vi "protocol_combined.vi"() -> ()   [LabVIEW 2015]
uses:
  dxl_x86_c.lvlib/dxl_x86_c.lvlib
panel:
  out "protocol_version2":dbl=2.0
  in  "value : MX (dial)\ngoal position 1":u16(knob)
  in  "ADDR_MX_\nPRESENT_POSITION":u16=36
  in  "ADDR_MX_\nGOAL_POSITION":u16=30
  in  "ADDR_MX_\nTORQUE_ENABLE":u16=24
  out "value : PRO (knob)\npresent position 2":i32(knob) scale=150000.0..-150000.0
  in  "dynamixe2_id":u8=2
  in  "device_name1":string="COM1"
  in  "ADDR_PRO_\nPRESENT_POSITION":u16=611
  in  "ADDR_PRO_\nGOAL_POSITION":u16=596
  in  "ADDR_PRO_\nTORQUE_ENABLE":u16=562
  out "protocol_version1":dbl=1.0
  out "value : MX (knob)\npresent position 1":u16(knob)
  in  "terminate":bool
  out "port_num":i32
  in  "value : PRO (dial)\ngoal position 2":i32(knob) scale=150000.0..-150000.0
  in  "dynamixel1_id":u8=1
  in  "baud_rate":i32=1000000
  # "protocol_combined.vi\n\nCreated on: 2016. 6. 13\nAuthor: Ryu Woon Jung (Leon)\n\n*********     Protocol Combined Example      *********\n\n\nAvailable Dynamixel model on this example : All models using Protocol 1.0 and 2.0\nThis example is designed for using a Dynamixel MX-28, a Dynamixel PRO 54-200 and an USB2DYNAMIXEL\nTo use another Dynamixel model, such as X series, see their details in E-Manual(support.robotis.com) \n   and edit \"numeric control\"s seen left with \"Edit Text\" tool.\nBe sure that properties of Dynamixel MX and PRO are already set as %% MX - ID : 1 / Baudnum : 1 (Baudrate : 1000000) , PRO - ID : 1 / Baudnum : 3 (Baudrate : 1000000)\n\nBe aware that:\nThis example configures two different control tables (especially, if it uses Dynamixel and Dynamixel PRO). It may modify critical Dynamixel parameter on the control table, if Dynamixels have wrong ID.\n\n\n1. Run example by click above \"Run\" button (below \"Edit\" menu).\n2. Drag \"dial\" then you may see the Dynamixel and \"knob\"s rotating\n3. To finish the example, press \"terminate\" button."
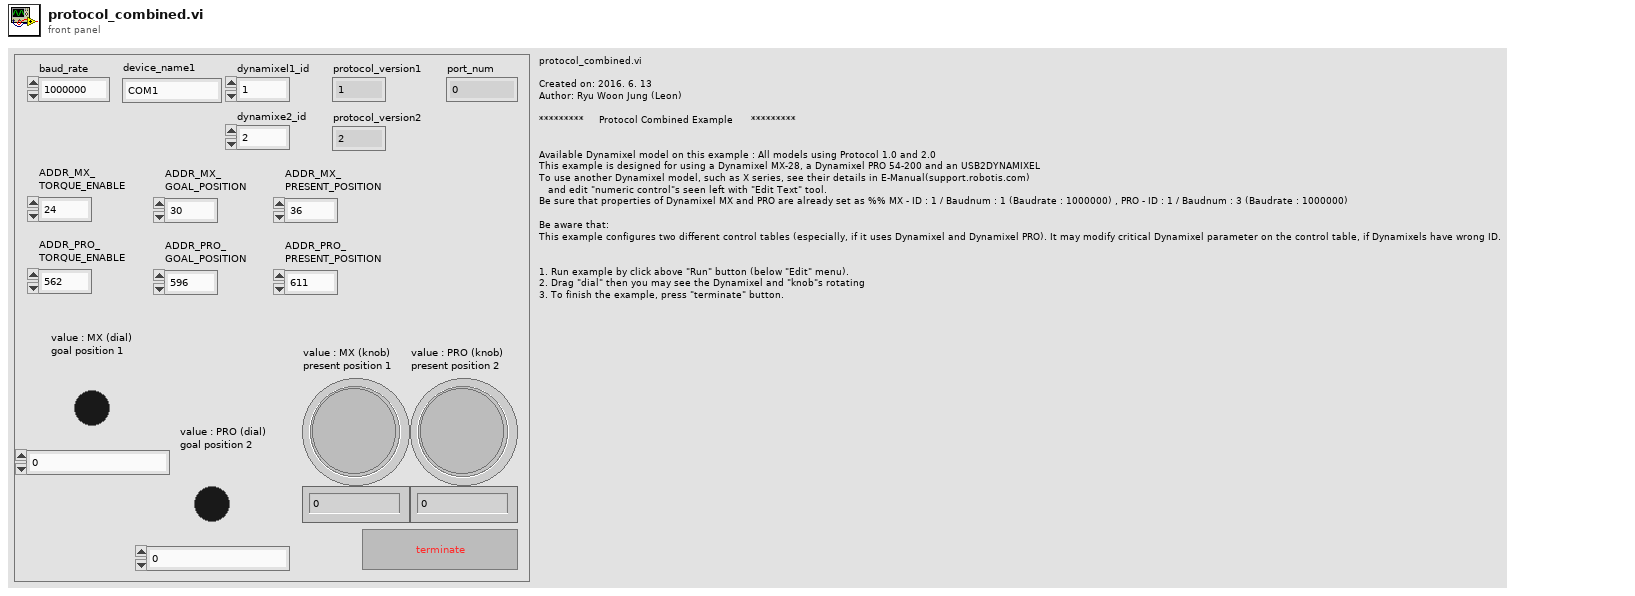
[diagram p1: front panel]
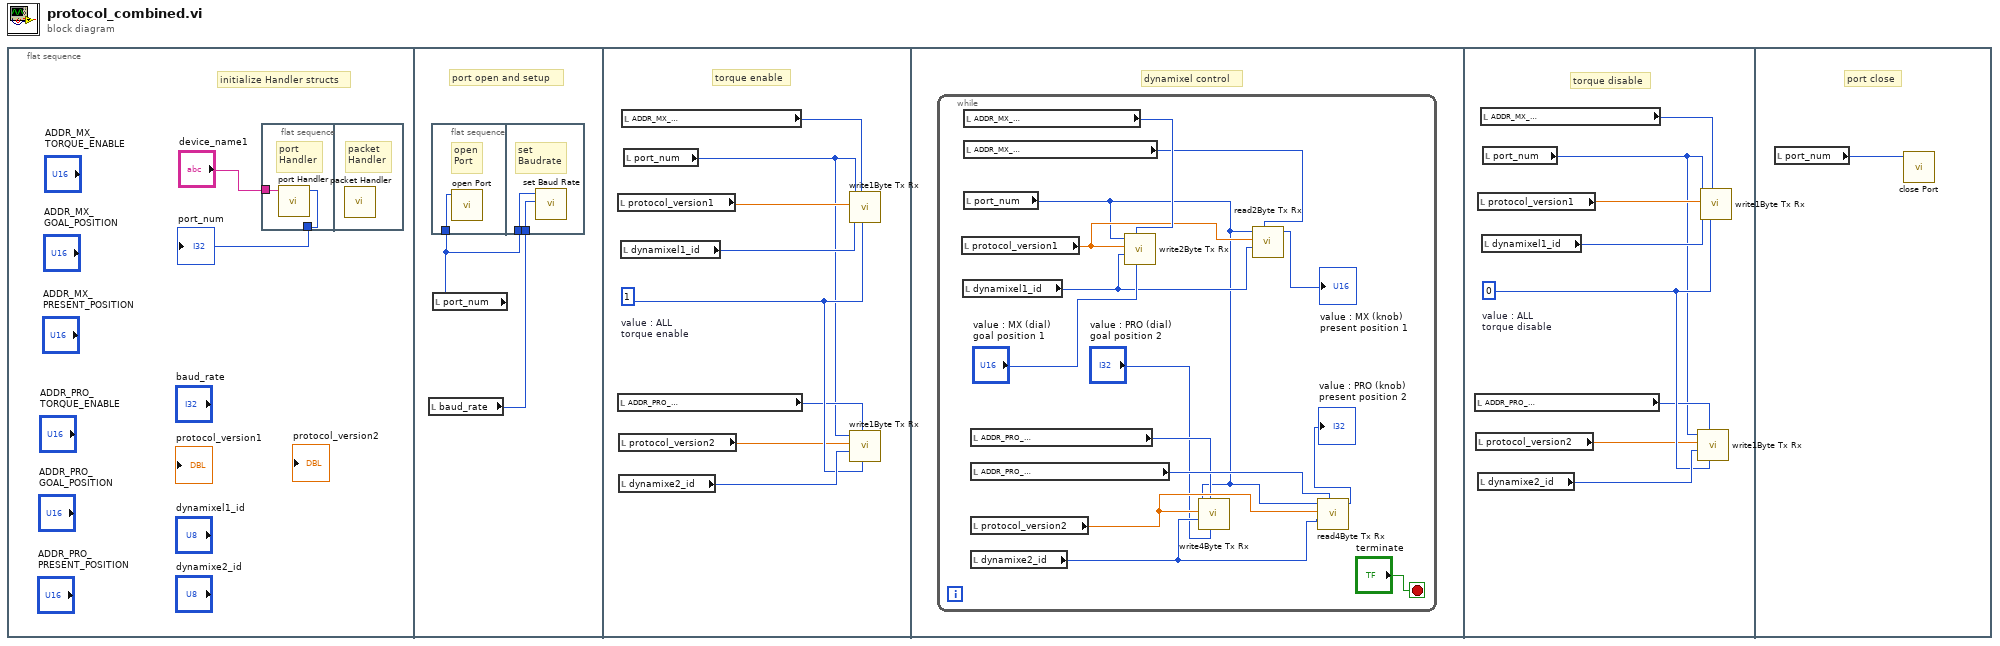
[diagram p0: block diagram]
diagram:
  n1 = flat-sequence {
    frame #0 {
      # "initialize Handler structs"
      n2 = flat-sequence {
        tunnel: "device_name1" -> [w4]
        tunnel: [w3] -> w1
        frame #0 {
          # "port\nHandler"
          n3 = call "port Handler.vi"("port_name"=w4) -> ("function return"=w3:i32)  [unwired: 10 in]
        }
        frame #1 {
          # "packet\nHandler"
          n4 = call "packet Handler.vi"() -> ()  [unwired: 12 in]
        }
      }
      "port_num" <- w1
    }
    frame #1 {
      # "port open and setup"
      n5 = local read "baud_rate"() -> (w5:i32)
      n6 = flat-sequence {
        tunnel: w6 -> [w7]
        tunnel: w6 -> [w9]
        tunnel: w5 -> [w8]
        frame #0 {
          # "open\nPort"
          n7 = call "open Port.vi"("port_num"=w7) -> ()  [unwired: 10 in, 1 out]
        }
        frame #1 {
          # "set\nBaudrate"
          n8 = call "set Baud Rate.vi"("baudrate"=w8, "port_num"=w9) -> ()  [unwired: 9 in, 1 out]
        }
      }
      n9 = local read "port_num"() -> (w6:i32)
    }
    frame #2 {
      w13 = 1  # value : ALL torque enable
      # "torque enable"
      n10 = local read "protocol_version1"() -> (w15:dbl)
      n11 = local read "ADDR_PRO_\nTORQUE_ENABLE"() -> (w12:u16)
      n12 = local read "protocol_version2"() -> (w10:dbl)
      n13 = local read "dynamixe2_id"() -> (w14:u8)
      n14 = local read "dynamixel1_id"() -> (w17:u8)
      n15 = local read "ADDR_MX_\nTORQUE_ENABLE"() -> (w16:u16)
      n16 = local read "port_num"() -> (w11:i32)
      n17 = call "write1Byte Tx Rx.vi"("data"=w13, "address"=w16, "id"=w17, "protocol_version"=w15, "port_num"=w11) -> ()  [unwired: 7 in]
      n18 = call "write1Byte Tx Rx.vi"("data"=w13, "address"=w12, "id"=w14, "protocol_version"=w10, "port_num"=w11) -> ()  [unwired: 7 in]
    }
    frame #3 {
      # "dynamixel control"
      n19 = while {
        stop <- "terminate" stop-if-true
        n20 = local read "protocol_version1"() -> (w20:dbl)
        n21 = local read "dynamixel1_id"() -> (w19:u8)
        n22 = local read "ADDR_MX_\nGOAL_POSITION"() -> (w28:u16)
        n23 = local read "ADDR_MX_\nPRESENT_POSITION"() -> (w22:u16)
        n24 = local read "port_num"() -> (w18:i32)
        n25 = local read "ADDR_PRO_\nGOAL_POSITION"() -> (w25:u16)
        n26 = local read "ADDR_PRO_\nPRESENT_POSITION"() -> (w26:u16)
        n27 = local read "protocol_version2"() -> (w27:dbl)
        n28 = local read "dynamixe2_id"() -> (w29:u8)
        n29 = call <userlib>:"write2Byte Tx Rx.vi"("data"="value : MX (dial)\ngoal position 1", "address"=w28, "id"=w19, "protocol_version"=w20, "port_num"=w18) -> ()  [unwired: 7 in]
        n30 = call "write4Byte Tx Rx.vi"("data"="value : PRO (dial)\ngoal position 2", "address"=w25, "id"=w29, "protocol_version"=w27, "port_num"=w18) -> ()  [unwired: 7 in]
        n31 = call <userlib>:"read2Byte Tx Rx.vi"("address"=w22, "id"=w19, "protocol_version"=w20, "port_num"=w18) -> ("function return"=→"value : MX (knob)\npresent position 1":u16)  [unwired: 7 in]
        n32 = call "read4Byte Tx Rx.vi"("address"=w26, "id"=w29, "protocol_version"=w27, "port_num"=w18) -> ("function return"=→"value : PRO (knob)\npresent position 2":u32)  [unwired: 7 in]
      }
    }
    frame #4 {
      w35 = 0  # value : ALL torque disable
      # "torque disable"
      n33 = local read "ADDR_PRO_\nTORQUE_ENABLE"() -> (w34:u16)
      n34 = local read "protocol_version2"() -> (w32:dbl)
      n35 = local read "protocol_version1"() -> (w37:dbl)
      n36 = local read "dynamixe2_id"() -> (w36:u8)
      n37 = local read "ADDR_MX_\nTORQUE_ENABLE"() -> (w38:u16)
      n38 = local read "dynamixel1_id"() -> (w39:u8)
      n39 = local read "port_num"() -> (w33:i32)
      n40 = call "write1Byte Tx Rx.vi"("data"=w35, "address"=w34, "id"=w36, "protocol_version"=w32, "port_num"=w33) -> ()  [unwired: 7 in]
      n41 = call "write1Byte Tx Rx.vi"("data"=w35, "address"=w38, "id"=w39, "protocol_version"=w37, "port_num"=w33) -> ()  [unwired: 7 in]
    }
    frame #5 {
      # "port close"
      n42 = local read "port_num"() -> (w40:i32)
      n43 = call "close Port.vi"("port_num"=w40) -> ()  [unwired: 11 in]
    }
  }
